vi "FourFlippingCoins.vi"() -> ()   [LabVIEW 2013]
panel:
  out "Histogram":dynamicdata(graph)
  in  "Total Number of Trials":sgl
  out "Number of Heads":dbl
  out "Coin 4":bool
  out "Coin 3":bool
  out "Coin 2":bool
  out "Coin 1":bool
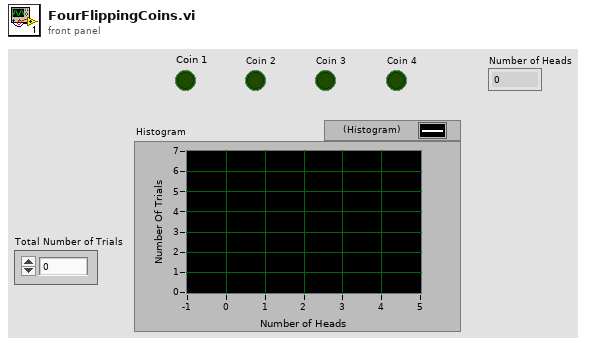
[diagram p1: front panel]
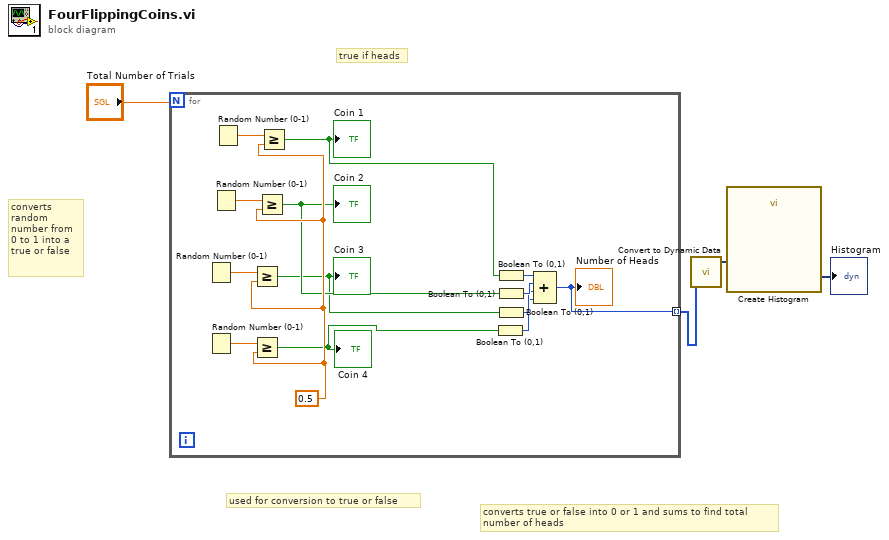
[diagram p0: block diagram]
diagram:
  # "true if heads"
  # "converts true or false into 0 or 1 and sums to find total\nnumber of heads"
  # "used for conversion to true or false"
  # "converts random number from 0 to 1 into a true or false"
  n1 = for {
    N: "Total Number of Trials" -> [_]
    tunnel: [w9] -> w3 mode=indexing
    w14 = 0.5
    n2 = Random Number (0-1)() -> (number: 0 to 1=w16:dbl)
    n3 = Random Number (0-1)() -> (number: 0 to 1=w15:dbl)
    n4 = Random Number (0-1)() -> (number: 0 to 1=w17:dbl)
    n5 = Random Number (0-1)() -> (number: 0 to 1=w18:dbl)
    n6 = Greater Or Equal?(x=w16, y=w14) -> (x >= y?=w11:bool)
    "Coin 3" <- w11
    n7 = Greater Or Equal?(x=w15, y=w14) -> (x >= y?=w10:bool)
    "Coin 4" <- w10
    n8 = Greater Or Equal?(x=w17, y=w14) -> (x >= y?=w12:bool)
    "Coin 2" <- w12
    n9 = Greater Or Equal?(x=w18, y=w14) -> (x >= y?=w13:bool)
    "Coin 1" <- w13
    n10 = Boolean To (0,1)(Boolean=w10) -> (0, 1=w5:i16)
    n11 = Boolean To (0,1)(Boolean=w13) -> (0, 1=w8:i16)
    n12 = Boolean To (0,1)(Boolean=w12) -> (0, 1=w7:i16)
    n13 = Boolean To (0,1)(Boolean=w11) -> (0, 1=w6:i16)
    n14 = Compound Arithmetic op=ADD(w8, w7, w6, w5) -> (w9:i16)
    "Number of Heads" <- w9
  }
  n15 = call "Convert to Dynamic Data"("Array"=w3) -> ("Dynamic Data Type"=w2:dynamicdata)  [unwired: 3 in]
  n16 = call "Create Histogram"("Signal"=w2) -> ("Histogram"=→"Histogram":dynamicdata)  [unwired: 9 in, 1 out]
